vi "Example_OE1022D Control.vi"() -> ()   [LabVIEW 2019]
uses:
  <vilib>/Utility/error.llb/DialogType.ctl
panel:
  in  "Sample count":u32
  out "Zero Data?":bool
  in  "buffer":u8
  out "Queue out":errorcluster caption="error out"
  out "Queue output":refnum<queue>
  in  "Timeout":u32=1000
  out "A_Gain Overlaod":bool
  out "B_Gain Overlaod":bool
  out "B_Input Overlaod":bool
  out "B_PLL Lock":bool
  out "B_Freq":dbl
  out "B_xita":dbl
  out "B_R":dbl
  in  "Remote Mode":u16(ring) items=["USB", "RS232", "GPIB"]
  out "A_Freq":dbl
  out "A_xita":dbl
  out "A_R":dbl
  out "A_Input Overlaod":bool
  out "A_PLL Lock":bool
  out "Error":string
  out "Serial Versions":string
  in  "Table":T1(tab) caption="选项卡控件"
  in  "OE1022D_Configure Input Filter":T2={"Input Source"=0, "Input Shield Grounding "=0, "Input Coupling "=0, "Input Notch Filter "=0, "Channel"=1} {"Channel" items=["A"=1, "B"=2]; "Input Notch Filter" items=["None"=0, "50Hz"=1, "100Hz"=3, "Both"=2]; "Input Coupling" items=["AC", "DC"]; "Input Shield Grounding" items=["Float", "Ground"]; "Input Source" items=["A", "B", "I-1M", "I-100M"]}
  in  "OE1022D_Configure Ref Phase":T3={"Sweep Mode"=0, "Start Frequency"=1000.0, "Stop Frequency"=0.001, "Linear Step Frequency"=1000.0, "Log Step Percent"=10.0, "Step Time(ms)"=1000, "Sweep Run Mode"=0, "Internal Frequency"=1000.0, "Phase  (degree)"=0.0, "External Ref Trigger"=0, "Reference Source"=0, "Channel"=1} {"Channel" items=["A"=1, "B"=2]; "Reference Source" items=["External", "Internal", "Internal Sweep", "Channel-A"]; "External Ref Trigger" items=["TTL Rising Edge", "TTL Falling Edge", "Sine Zero Crossing"]; "Phase  (degree)" min=-180.0 max=180.0 format="%#.2g"; "Internal Frequency" min=0.001 max=102000.0 format="%#.3f"; "Sweep Run Mode" items=["Stop", "Singal", "Loop"]; "Step Time(ms)" min=1 max=100000; "Log Step Percent" min=0.0 max=100.0 format="%#.2g"; "Linear Step Frequency" min=0.001 max=102000.0 format="%#.3f"; "Stop Frequency" min=0.001 max=102000.0 format="%#.3f"; "Start Frequency" min=0.001 max=102000.0 format="%#.3f"; "Sweep Mode" items=["Linear", "Log"]}
  in  "OE1022D_Configure Sens and Filter":T4={"Dynamic Reserve"=1, "Sensitivity "=24, "Time Constant "=9, "Low Pass Filter Slope "=1, "Enable Sync Filter "=0, "Channel"=1} {"Channel" items=["A"=1, "B"=2]; "Enable Sync Filter" items=["OFF", "ON"]; "Low Pass Filter Slope" items=["6 dB/oct", "12 dB/oct", "18 db/oct", "24 dB/oct"]; "Time Constant" items=["10 us", "30 us", "100 us", "300 us", "1 ms", "3 ms", "10 ms", "30 ms", "100 ms", "300 ms", "1 s", "3 s", "10 s", "30 s", "100 s", "300 s", "1 ks", "3 ks"]; "Sensitivity" items=["1 nV/fA", "2 nV/fA", "5 nV/fA", "10 nV/fA", "20 nV/fA", "50 nV/fA", "100 nV/fA", "200 nV/fA", "500 nV/fA", "1 uV/pA", "2 uV/pA", "5 uV/pA", "10 uV/pA", "20 uV/pA", "50 uV/pA", "100 uV/pA", "200 uV/pA", "500 uV/pA", "1 mV/nA", "2 mV/nA", "5 mV/nA", "10 mV/nA", "20 mV/nA", "50 mV/nA", "100 mV/nA", "200 mV/nA", "500 mV/nA", "1 V/uA"]; "Dynamic Reserve" items=["Low Noise", "Normal", "High Reserve"]}
  in  "OE1022D_Configure Channel Out":T5={"CH1 Speed"=0, "CH2 Offset(%)"=0.0, "CH1 Offset(%)"=0.0, "CH2 Expand"=1.0, "CH1 Expand"=1.0, "CH1"=0, "CH2"=0, "AUX OUT1"=1.0, "AUX OUT2"=1.0, "CH2 Speed"=0} {"CH2 Speed" items=["Slow", "Fast"]; "AUX OUT2" min=-10.0 max=10.0 format="%#.3g"; "AUX OUT1" min=-10.0 max=10.0 format="%#.3g"; "CH2" items=["A-R", "A-X", "A-Y", "A-Theta", "A-Rh1", "A-Xh1", "A-Yh1", "A-Theta h1", "A-Rh2", "A-Xh2", "A-Yh2", "A-Theta h2", "A-Noise", "A-E1", "A-E2", "A-E3", "A-E4", "B-R", "B-X", "B-Y", "B-Theta", "B-Rh1", "B-Xh1", "B-Yh1", "B-Theta h1", "B-Rh2", "B-Xh2", "B-Yh2", "B-Theta h2", "B-Noise", "B-E1", "B-E2", "B-E3", "B-E4", "AUX OUT"]; "CH1" items=["A-R", "A-X", "A-Y", "A-Theta", "A-Rh1", "A-Xh1", "A-Yh1", "A-Theta h1", "A-Rh2", "A-Xh2", "A-Yh2", "A-Theta h2", "A-Noise", "A-E1", "A-E2", "A-E3", "A-E4", "B-R", "B-X", "B-Y", "B-Theta", "B-Rh1", "B-Xh1", "B-Yh1", "B-Theta h1", "B-Rh2", "B-Xh2", "B-Yh2", "B-Theta h2", "B-Noise", "B-E1", "B-E2", "B-E3", "B-E4", "AUX OUT"]; "CH1 Expand" min=1.0 max=256.0 format="%#_3g"; "CH2 Expand" min=1.0 max=256.0 format="%#_3g"; "CH1 Offset(%)" min=-100.0 max=100.0 format="%#_5g"; "CH2 Offset(%)" min=-100.0 max=100.0 format="%#_5g"; "CH1 Speed" items=["Slow", "Fast"]}
  in  "OE1022D_Configure Sine Out":T6={"Start Value"=1.0, "Sine Output Amplitude "=1.0, "Stop Valve"=5.0, "Sine Step Valve"=1.0, "Step Time "=1000, "Sine Step Percent"=10.0, "SineOut Mode"=0, "Sine Run Mode"=0, "Channel"=1, "Sine Output DC "=1.0} {"Sine Output DC" min=-10.0 max=10.0 format="%#.3f"; "Channel" items=["A"=1, "B"=2]; "Sine Run Mode" items=["Stop", "Single", "Loop"]; "SineOut Mode" items=["Fixed", "Linear", "Log", "DC"]; "Sine Step Percent" min=0.0 max=100.0 format="%#.3g"; "Step Time" min=1 max=100000; "Sine Step Valve" min=0.001 max=5.0 format="%#.3g"; "Stop Valve" min=0.001 max=5.0 format="%#.3g"; "Sine Output Amplitude" min=0.001 max=5.0 format="%#.3g"; "Start Value" min=0.001 max=5.0 format="%#.3g"}
  in  "OE1022D_Configure Harmonic":T7={"Harmonic 1"=1, "Harmonic 2"=1, "Channel"=1} {"Channel" items=["A"=1, "B"=2]; "Harmonic 2" min=1 max=32767; "Harmonic 1" min=1 max=32767}
  in  "OE1022D_Configure Sample":T8={"Trigger Mode"=0, "Sample Mode"=0, "Buffer 1"=0, "Buffer 2"=1, "Buffer 3"=2, "Sample Time(ms)"=100, "Length"=50, "Buffer 4"=3, "Channel"=1, "Sample State"=0} {"Sample State" items=["Start", "Pause", "Stop and Clear"]; "Channel" items=["A"=1, "B"=2]; "Buffer 4" items=["R", "X", "Y", "Theta", "Rh1", "Xh1", "Yh1", "Theta h1", "Rh2", "Xh2", "Yh2", "Theta h2", "Noise", "A1", "A2", "A3", "A4", "Freq", "C1", "C2"]; "Length" min=1 max=16384; "Sample Time(ms)" min=1 max=100000; "Buffer 3" items=["R", "X", "Y", "Theta", "Rh1", "Xh1", "Yh1", "Theta h1", "Rh2", "Xh2", "Yh2", "Theta h2", "Noise", "A1", "A2", "A3", "A4", "Freq", "C1", "C2"]; "Buffer 2" items=["R", "X", "Y", "Theta", "Rh1", "Xh1", "Yh1", "Theta h1", "Rh2", "Xh2", "Yh2", "Theta h2", "Noise", "A1", "A2", "A3", "A4", "Freq", "C1", "C2"]; "Buffer 1" items=["R", "X", "Y", "Theta", "Rh1", "Xh1", "Yh1", "Theta h1", "Rh2", "Xh2", "Yh2", "Theta h2", "Noise", "A1", "A2", "A3", "A4", "Freq", "C1", "C2"]; "Sample Mode" items=["Single", "Loop"]; "Trigger Mode" items=["Int", "Ext"]}
  in  "OE1022D_Configure Equation":T9={"A"=0, "B"=18, "C"=19, "E"=1, "C1"=0.0, "C2"=0.0, "Channel"=1} {"Channel" items=["A"=1, "B"=2]; "C2" min=-10.0 max=10.0 format="%.3f"; "C1" min=-10.0 max=10.0 format="%.3f"; "E" items=["1"=1, "2"=2, "3"=3, "4"=4]; "C" items=["R", "X", "Y", "Theta", "Rh1", "Xh1", "Yh1", "Theta h1", "Rh2", "Xh2", "Yh2", "Theta h2", "Noise", "A1", "A2", "A3", "A4", "Freq", "C1", "C2"]; "B" items=["R", "X", "Y", "Theta", "Rh1", "Xh1", "Yh1", "Theta h1", "Rh2", "Xh2", "Yh2", "Theta h2", "Noise", "A1", "A2", "A3", "A4", "Freq", "C1", "C2"]; "A" items=["R", "X", "Y", "Theta", "Rh1", "Xh1", "Yh1", "Theta h1", "Rh2", "Xh2", "Yh2", "Theta h2", "Noise", "A1", "A2", "A3", "A4", "Freq", "C1", "C2"]}
  in  "OE1022D_Auto Setting":T10={"Auto Gain"=FALSE, "Auto Reserve"=FALSE, "Auto Phase"=FALSE, "Auto Scale"=FALSE, "Channel"=1} {"Channel" items=["A"=1, "B"=2]}
  in  "Save Button":bool
  in  "file path":path
  in  "Sample Rate":dbl=0.1 min=0.1 max=100.0
  out "Status":string
  in  "Connect":bool
  in  "VISA resource name":refnum<visa-resource-name>
  in  "Baud rate (921600)":u32=921600
  # "Tel          :   +86-020-84133345\nWebsite  :   www.ssi-instrument.com\nE-mail     :   support@si-instrument.com"
  # "X"
  # "="
  # "______________________________________________________"
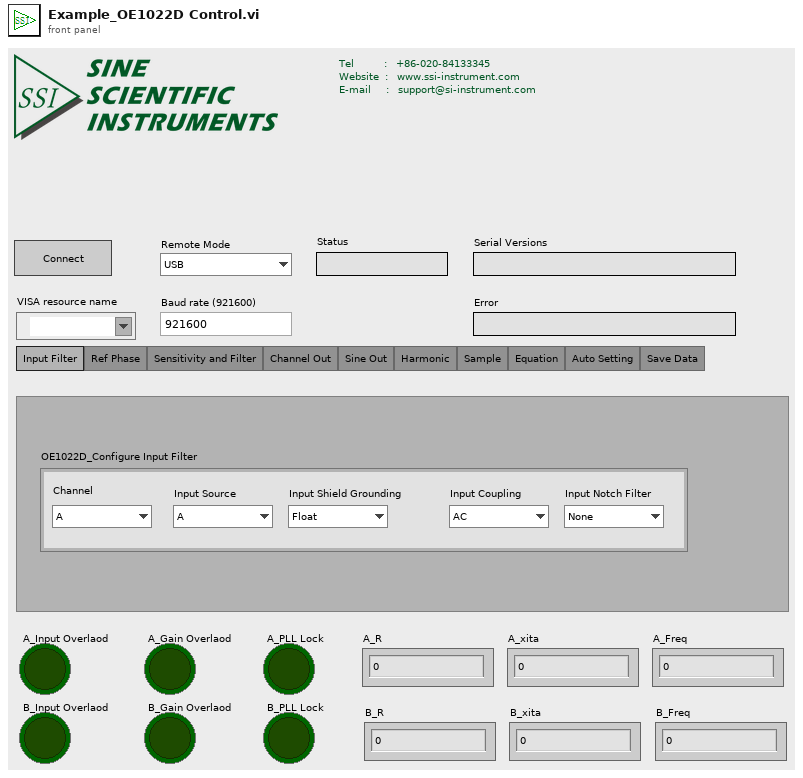
[diagram p1: front panel]
types:
  T1 = enum32{"Input Filter", "Ref Phase", "Sensitivity and Filter", "Channel Out", "Sine Out", "Harmonic", "Sample", "Equation", "Auto Setting", "Save Data"}
  T2 = cluster{"Input Source":u16, "Input Shield Grounding ":u16, "Input Coupling ":u16, "Input Notch Filter ":u16, "Channel":u16}
  T3 = cluster{"Sweep Mode":u16, "Start Frequency":dbl, "Stop Frequency":dbl, "Linear Step Frequency":dbl, "Log Step Percent":dbl, "Step Time(ms)":u32, "Sweep Run Mode":u16, "Internal Frequency":dbl, "Phase  (degree)":dbl, "External Ref Trigger":u16, "Reference Source":u16, "Channel":u16}
  T4 = cluster{"Dynamic Reserve":u16, "Sensitivity ":u16, "Time Constant ":u8, "Low Pass Filter Slope ":u8, "Enable Sync Filter ":u16, "Channel":u16}
  T5 = cluster{"CH1 Speed":u16, "CH2 Offset(%)":dbl, "CH1 Offset(%)":dbl, "CH2 Expand":dbl, "CH1 Expand":dbl, "CH1":u16, "CH2":u16, "AUX OUT1":dbl, "AUX OUT2":dbl, "CH2 Speed":u16}
  T6 = cluster{"Start Value":dbl, "Sine Output Amplitude ":dbl, "Stop Valve":dbl, "Sine Step Valve":dbl, "Step Time ":u32, "Sine Step Percent":dbl, "SineOut Mode":u8, "Sine Run Mode":u8, "Channel":u16, "Sine Output DC ":dbl}
  T7 = cluster{"Harmonic 1":u16, "Harmonic 2":u16, "Channel":u16}
  T8 = cluster{"Trigger Mode":u16, "Sample Mode":u16, "Buffer 1":u16, "Buffer 2":u16, "Buffer 3":u16, "Sample Time(ms)":u32, "Length":u16, "Buffer 4":u16, "Channel":u16, "Sample State":u16}
  T9 = cluster{"A":u16, "B":u16, "C":u16, "E":u16, "C1":dbl, "C2":dbl, "Channel":u16}
  T10 = cluster{"Auto Gain":bool, "Auto Reserve":bool, "Auto Phase":bool, "Auto Scale":bool, "Channel":u16}
  T11 = enum16{"OE1022", "OE1022D", "OE1201", "OE2031&OE2041", "OE1311&OE1351"}
  T12 = cluster{"PLL Lock(1: External Lock)":bool, "Input Overlaod":bool, "Gain Overlaod":bool}
  T13 = cluster{"A_X":dbl, "A_Y":dbl, "A_R":dbl, "A_θ":dbl, "A_Frequency":dbl, "A_Noise":dbl, "A_Xh1":dbl, "A_Yh1":dbl, "A_Rh1":dbl, "A_θh1":dbl, "A_Xh2":dbl, "A_Yh2":dbl, "A_Rh2":dbl, "A_θh2":dbl, "B_X":dbl, "B_Y":dbl, "B_R":dbl, "B_θ":dbl, "B_Frequency":dbl, "B_Noise":dbl, "B_Xh1":dbl, "B_Yh1":dbl, "B_Rh1":dbl, "B_θh1":dbl, "B_Xh2":dbl, "B_Yh2":dbl, "B_Rh2":dbl, "B_θh2":dbl, "A1":dbl, "A2":dbl, "A3":dbl, "A4":dbl}
  T14 = cluster{"A_PLL&Overload":cluster{"PLL Lock(1: External Lock)":bool, "Input Overlaod":bool, "Gain Overlaod":bool}, "B_PLL&Overload":cluster{"PLL Lock(1: External Lock)":bool, "Input Overlaod":bool, "Gain Overlaod":bool}}
  T15 = typedef "DialogType.ctl" = u16
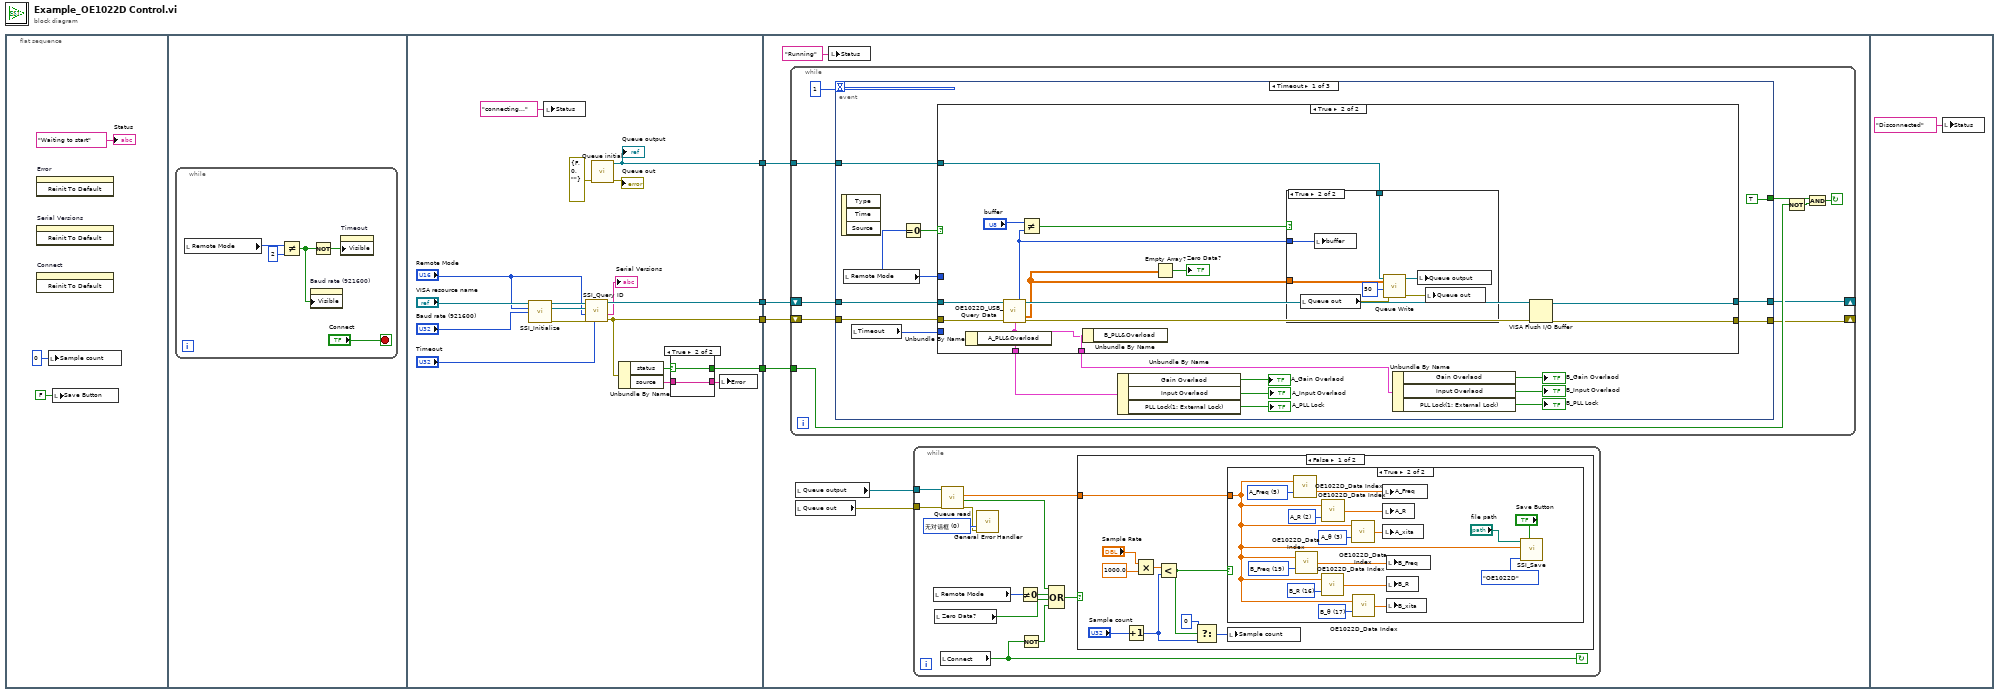
[diagram p0: block diagram]
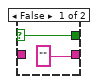
[diagram p2: hidden frame]
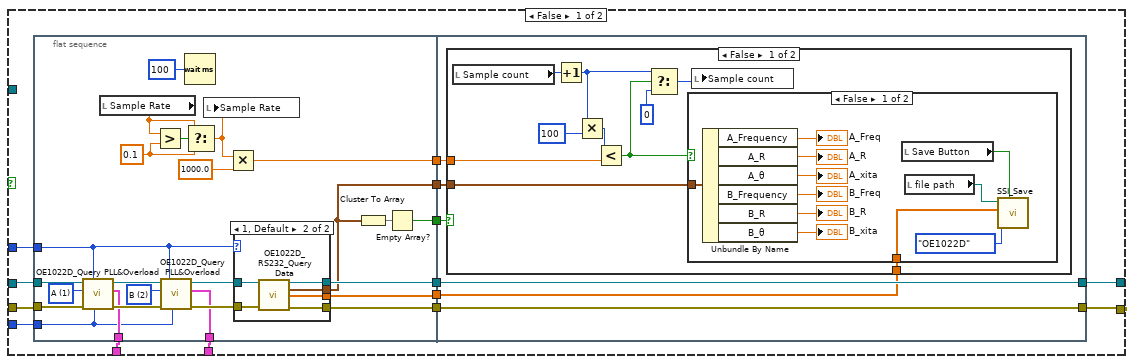
[diagram p5: hidden frame]
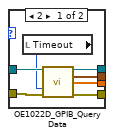
[diagram p6: hidden frame]
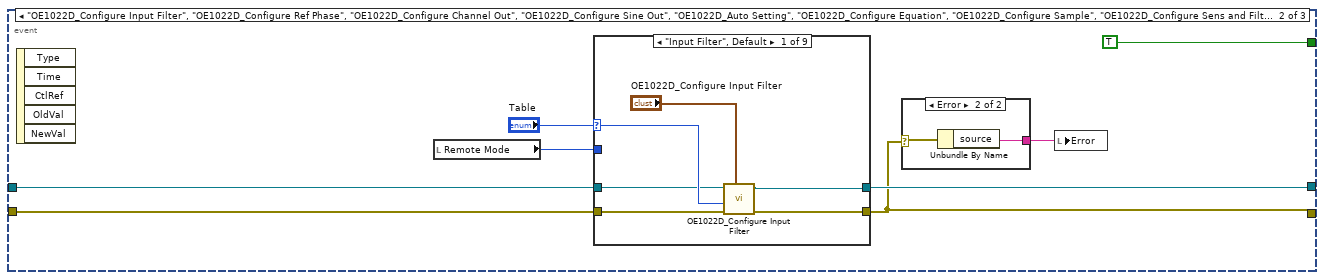
[diagram p10: hidden frame]
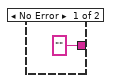
[diagram p11: hidden frame]
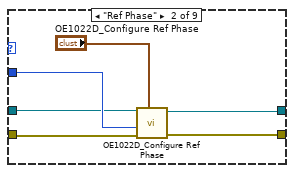
[diagram p12: hidden frame]
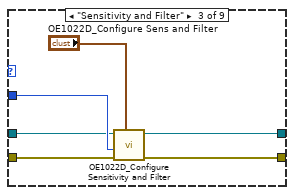
[diagram p13: hidden frame]
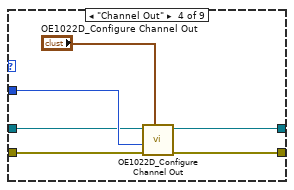
[diagram p14: hidden frame]
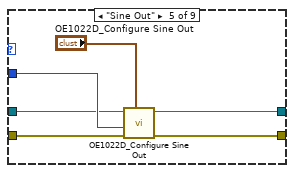
[diagram p15: hidden frame]
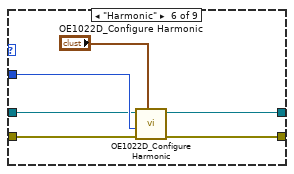
[diagram p16: hidden frame]
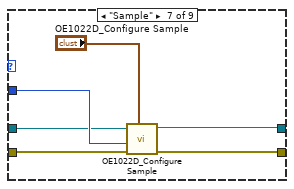
[diagram p17: hidden frame]
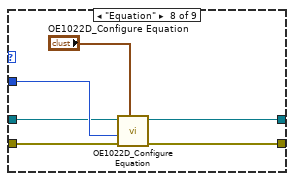
[diagram p18: hidden frame]
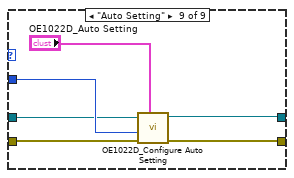
[diagram p19: hidden frame]
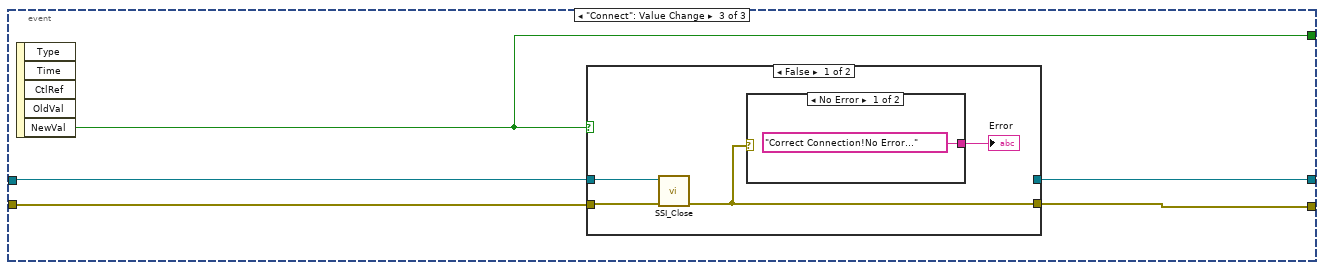
[diagram p20: hidden frame]
diagram:
  n1 = flat-sequence {
    tunnel: [w24] -> w4
    tunnel: [w19] -> w3
    tunnel: [w18] -> w2
    tunnel: [w13] -> w1
    tunnel: w4 -> [w40]
    tunnel: w3 -> [w39]
    tunnel: w2 -> [w38]
    tunnel: w1 -> [w37]
    frame #0 {
      n2 = invoke on="Error" class="Str" method="Reinit To Default"() -> ()  [unwired: 3 in, 3 out]
      n3 = invoke on="Serial Versions" class="Str" method="Reinit To Default"() -> ()  [unwired: 3 in, 3 out]
      n4 = invoke on="Connect" class="Bool (严格)" method="Reinit To Default"() -> ()  [unwired: 3 in, 3 out]
      n5 = local write "Sample count"(u32 0 ("Sample count")) -> ()
      n6 = local write "Save Button"(FALSE ("Save Button")) -> ()
      "Status" <- "Waiting to start" ("status")
    }
    frame #1 {
      n7 = while {
        stop <- "Connect" stop-if-true
        n8 = local read "Remote Mode"() -> (w11:u16)
        n9 = Not Equal?(x=w11, y=u16 2) -> (x != y?=w9:bool)
        n10 = property on="Baud rate (921600)" class="DigNum (strict)"("Visible"=w9) -> ()  [unwired: 2 in, 2 out]
        n11 = Not(x=w9) -> (.not. x?=w8:bool)
        n12 = property on="Timeout" class="DigNum (strict)"("Visible"=w8) -> ()  [unwired: 2 in, 2 out]
      }
    }
    frame #2 {
      n13 = call "SSI_Initialize.vi"("VISA resource name"="VISA resource name", "Remote Mode"="Remote Mode", "baud rate (921600)"="Baud rate (921600)") -> ("VISA resource name out"=w28:refnum<visa-resource-name>, "connection ID(Ethernet)"=w27:refnum<k5>, "error out"=w26:errorcluster)  [unwired: 10 in]
      n14 = local write "Status"("connecting..." ("status")) -> ()
      n15 = call "SSI_Query ID.vi"("Timeout"="Timeout", "Error in (no error)"=w26, "Remote Mode"="Remote Mode", "Connection ID in"=w27, "VISA resource name"=w28) -> ("Error out"=w19:errorcluster, "Read Buffer"=→"Serial Versions":string, "VISA resource  out"=w24:refnum<visa-resource-name>)  [unwired: 3 in, 1 out]
      n16 = call "Queue initial.vi"("Error in (no error)"=errorcluster {"status"=FALSE, "code"=0, "source"=""}) -> ("Error out"=→"Queue out":errorcluster, "Queue output"=w13:refnum<queue>)  [unwired: 9 in]
      "Queue output" <- w13
      n17 = Unbundle By Name(w19) -> ("status"=w21:bool, "source"=w20:string)
      n18 = case shown="True" w21 {
        selector: w21 -> [w32 w34]
        tunnel: [w32 w34] -> w18
        tunnel: ["" w33] -> w17
        tunnel: w20 -> [_ w33]
        frame False {
        }
        frame True {
        }
      }
      n19 = local write "Error"(w17) -> ()
    }
    frame #3 {
      n20 = while {
        tunnel: w38 -> [w82]
        tunnel: w37 -> [w81]
        shift-right: [w79] -> _
        shift-left: w40 -> [w84]
        shift-right: [w80] -> _
        shift-left: w39 -> [w83]
        stop <- w86 continue-if-true
        n21 = event shown="[0] Timeout" {
          selector: _ -> [_ _ _]
          dyn-events: _ -> [_ _ _]
          timeout: 1 -> [_ _ _]
          tunnel: [TRUE ("Stop") TRUE ("Stop") w275] -> w85
          tunnel: [w105 w210 w276] -> w80
          tunnel: [w104 w213 w272] -> w79
          tunnel: w84 -> [w102 w208 w273]
          tunnel: w83 -> [w101 w207 w274]
          tunnel: w81 -> [w90 _ _]
          event Timeout {
            n22 = event-data() -> ()  [unwired: 1 in, 3 out]
            n23 = local read "Remote Mode"() -> (w92:u16)
            n24 = local read "Timeout"() -> (w89:u32)
            n25 = Equal To 0?(x=w92) -> (x = 0?=w91:bool)
            n26 = case shown="True" w91 {
              tunnel: [w119 w186] -> w105
              tunnel: [w118 w187] -> w104
              tunnel: w102 -> [w117 w192]
              tunnel: w101 -> [w116 w191]
              tunnel: [w115 w190] -> w100
              tunnel: [w114 w189] -> w99
              tunnel: w92 -> [w113 _]
              tunnel: w90 -> [_ w185]
              tunnel: w89 -> [w106 _]
              frame False {
                n27 = flat-sequence {
                  tunnel: [w131] -> w112
                  tunnel: [w132] -> w111
                  tunnel: [w140] -> w109
                  tunnel: [w122] -> w108
                  tunnel: [w130] -> w107
                  tunnel: [w127] -> w115
                  tunnel: [w126] -> w114
                  tunnel: w117 -> [w129]
                  tunnel: w116 -> [w128]
                  tunnel: w113 -> [w125]
                  tunnel: [w123] -> w110
                  tunnel: w106 -> [w120]
                  tunnel: w112 -> [w162]
                  tunnel: w111 -> [w163]
                  tunnel: [w163] -> w118
                  tunnel: [w162] -> w119
                  tunnel: w110 -> [w159]
                  tunnel: w109 -> [w158]
                  tunnel: w108 -> [w160]
                  tunnel: w107 -> [w161]
                  frame #0 {
                    w136 = u16 2 items=["A"=1, "B"=2] ("Channel")
                    w137 = u16 1 items=["A"=1, "B"=2] ("Channel")
                    w143 = 0.1 ("y")
                    n28 = call "OE1022D_Query PLL&Overload.vi"("Timeout"=w120, "Error in (no error)"=w128, "Remote Mode"=w125, "Channel"=w137, "VISA resource name"=w129) -> ("Error out"=w138:errorcluster, "OE1022D_Query PLL&Overload"=w127:T12, "VISA resource  out"=w135:refnum<visa-resource-name>)  [unwired: 3 in, 1 out]
                    n29 = local read "Sample Rate"() -> (w139:dbl)
                    n30 = Greater?(x=w139, y=w143) -> (0:w142:bool)
                    n31 = call "OE1022D_Query PLL&Overload.vi"("Timeout"=w120, "Error in (no error)"=w138, "Remote Mode"=w125, "Channel"=w136, "VISA resource name"=w135) -> ("Error out"=w134:errorcluster, "OE1022D_Query PLL&Overload"=w126:T12, "VISA resource  out"=w133:refnum<visa-resource-name>)  [unwired: 3 in, 1 out]
                    n32 = Wait (ms)(milliseconds to wait=u32 100 ("等待时间（毫秒）")) -> ()  [unwired: 1 out]
                    n33 = Select(t=w139, s=w142, f=w143) -> (s? t:f=w141:dbl)
                    n34 = local write "Sample Rate"(w141) -> ()
                    n35 = Multiply(x=w141, y=1000.0) -> (x*y=w140:dbl)
                    n36 = case shown="1, Default" w125 {
                      tunnel: w134 -> [w150 w157]
                      tunnel: w133 -> [w151 w156]
                      tunnel: [w149 w155] -> w132
                      tunnel: [w148 w154] -> w131
                      tunnel: [w147 w153] -> w130
                      tunnel: [w146 w152] -> w122
                      frame 2 {
                        n37 = local read "Timeout"() -> (w145:u32)
                        n38 = call "OE1022D_GPIB_Query Data.vi"("VISA resource name"=w151, "Timeout"=w145, "Error in (no error)"=w150) -> ("VISA resource  out"=w149:refnum<visa-resource-name>, "Parameter Values"=w146:T13, "Data Array"=w147:dbl[], "Error out"=w148:errorcluster)  [unwired: 8 in, 1 out]
                      }
                      frame 1, Default {
                        n39 = call "OE1022D_RS232_Query Data.vi"("VISA resource name"=w156, "Error in (no error)"=w157) -> ("VISA resource  out"=w155:refnum<visa-resource-name>, "Parameter Values"=w152:T13, "Data Array"=w153:dbl[], "Error out"=w154:errorcluster)  [unwired: 9 in, 1 out]
                      }
                    }
                    n40 = Cluster To Array(cluster=w122) -> (array=w124:dbl[])
                    n41 = Empty Array?(array=w124) -> (empty?=w123:bool)
                  }
                  frame #1 {
                    n42 = case shown="False" w159 {
                      tunnel: w161 -> [w173 _]
                      tunnel: w160 -> [w172 _]
                      tunnel: w158 -> [w168 _]
                      frame False {
                        n43 = local read "Sample count"() -> (w171:u32)
                        n44 = Increment(x=w171) -> (x+1=w167:u32)
                        n45 = Multiply(x=w167, y=u32 100) -> (x*y=w169:u32)
                        n46 = Less?(x=w169, y=w168) -> (x < y?=w165:bool)
                        n47 = Select(t=w167, s=w165, f=0) -> (s? t:f=w166:u32)
                        n48 = case shown="False" w165 {
                          tunnel: w172 -> [w175 _]
                          tunnel: w173 -> [w184 _]
                          frame False {
                            n49 = Unbundle By Name(w175) -> ("A_Frequency"=→"A_Freq":dbl, "A_R"=→"A_R":dbl, "A_θ"=→"A_xita":dbl, "B_Frequency"=→"B_Freq":dbl, "B_R"=→"B_R":dbl, "B_θ"=→"B_xita":dbl)
                            n50 = local read "Save Button"() -> (w182:bool)
                            n51 = local read "file path"() -> (w174:path)
                            n52 = call "SSI_Save.vi"("file path (dialog if empty)"=w174, "1D data"=w184, "Instrument Mode"=T11."OE1022D", "Save Button"=w182) -> ()  [unwired: 7 in]
                          }
                          frame True {
                          }
                        }
                        n53 = local write "Sample count"(w166) -> ()
                      }
                      frame True {
                      }
                    }
                  }
                }
              }
              frame True {
                n54 = call "OE1022D_USB_Query Data.vi"("VISA resource name"=w192, "Error in (no error)"=w191) -> ("Buffer Count"=w193:u8, "VISA resource  out"=w199:refnum<visa-resource-name>, "Total Date Array"=w194:dbl[][], "PLL&Overload"=w188:T14, "Error out"=w198:errorcluster)  [unwired: 6 in, 3 out]
                n55 = Unbundle By Name(w188) -> ("A_PLL&Overload"=w190:T12)
                n56 = Not Equal?(x="buffer", y=w193) -> (x != y?=w196:bool)
                n57 = Unbundle By Name(w188) -> ("B_PLL&Overload"=w189:T12)
                n58 = Empty Array?(array=w194) -> (empty?=→"Zero Data?":bool)
                n59 = case shown="True" w196 {
                  tunnel: w194 -> [_ w202]
                  tunnel: w193 -> [_ w201]
                  tunnel: w185 -> [_ w200]
                  frame False {
                  }
                  frame True {
                    n60 = local read "Queue out"() -> (w203:errorcluster)
                    n61 = local write "buffer"(w201) -> ()
                    n62 = call "Queue Write.vi"("Error in (no error)"=w203, "Group Count"=50, "Input Array"=w202, "Queue Input"=w200) -> ("Error out"=w204:errorcluster, "Queue output"=w205:refnum<queue>)  [unwired: 6 in]
                    n63 = local write "Queue output"(w205) -> ()
                    n64 = local write "Queue out"(w204) -> ()
                  }
                }
                n65 = VISA Flush I/O Buffer(VISA resource name=w199, error in (no error)=w198) -> (VISA resource name out=w187:refnum<visa-resource-name>, error out=w186:errorcluster)  [unwired: 1 in]
              }
            }
            n66 = Unbundle By Name(w100) -> ("Gain Overlaod"=→"A_Gain Overlaod":bool, "Input Overlaod"=→"A_Input Overlaod":bool, "PLL Lock(1: External Lock)"=→"A_PLL Lock":bool)
            n67 = Unbundle By Name(w99) -> ("Gain Overlaod"=→"B_Gain Overlaod":bool, "Input Overlaod"=→"B_Input Overlaod":bool, "PLL Lock(1: External Lock)"=→"B_PLL Lock":bool)
          }
          event "OE1022D_Configure Input Filter", "OE1022D_Configure Ref Phase", "OE1022D_Configure Channel Out", "OE1022D_Configure Sine Out", "OE1022D_Auto Setting", "OE1022D_Configure Equation", "OE1022D_Configure Sample", "OE1022D_Configure Sens and Filter", "OE1022D_Configure Harmonic": Value Change {
            n68 = event-data() -> ()  [unwired: 1 in, 5 out]
            n69 = local read "Remote Mode"() -> (w211:u16)
            n70 = case shown="\"Input Filter\", Default" "Table" {
              selector: "Table" -> [w223 _ _ _ _ _ _ _ _]
              tunnel: [w221 w228 w234 w240 w246 w251 w259 w262 w269] -> w213
              tunnel: [w220 w227 w235 w239 w247 w252 w258 w265 w268] -> w210
              tunnel: w211 -> [_ w226 w232 w238 w244 w250 w257 w264 w270]
              tunnel: w208 -> [w219 w225 w231 w237 w243 w249 w255 w261 w267]
              tunnel: w207 -> [w218 w224 w230 w236 w242 w248 w254 w260 w266]
              frame "Input Filter", Default {
                n71 = call "OE1022D_Configure Input Filter.vi"("OE1022D_Configure Input Filter"="OE1022D_Configure Input Filter", "Error in (no error)"=w218, "Remote Mode"=w223, "VISA resource name"=w219) -> ("Error out"=w220:errorcluster, "VISA resource  out"=w221:refnum<visa-resource-name>)  [unwired: 5 in, 1 out]
              }
              frame "Ref Phase" {
                n72 = call "OE1022D_Configure Ref Phase.vi"("OE1022D_Configure Ref Phase"="OE1022D_Configure Ref Phase", "Error in (no error)"=w224, "Remote Mode"=w226, "VISA resource name"=w225) -> ("Error out"=w227:errorcluster, "VISA resource  out"=w228:refnum<visa-resource-name>)  [unwired: 5 in, 1 out]
              }
              frame "Sensitivity and Filter" {
                n73 = call "OE1022D_Configure Sensitivity and Filter.vi"("OE1022D_Configure Sens and Filter"="OE1022D_Configure Sens and Filter", "Error in (no error)"=w230, "Remote Mode"=w232, "VISA resource name"=w231) -> ("Error out"=w235:errorcluster, "VISA resource  out"=w234:refnum<visa-resource-name>)  [unwired: 5 in, 1 out]
              }
              frame "Channel Out" {
                n74 = call "OE1022D_Configure Channel Out.vi"("OE1022D_Configure Channel Out"="OE1022D_Configure Channel Out", "Error in (no error)"=w236, "Remote Mode"=w238, "VISA resource name"=w237) -> ("Error out"=w239:errorcluster, "VISA resource  out"=w240:refnum<visa-resource-name>)  [unwired: 5 in, 1 out]
              }
              frame "Sine Out" {
                n75 = call "OE1022D_Configure Sine Out.vi"("OE1022D_Configure Sine Out"="OE1022D_Configure Sine Out", "Error in (no error)"=w242, "Remote Mode"=w244, "VISA resource name"=w243) -> ("Error out"=w247:errorcluster, "VISA resource  out"=w246:refnum<visa-resource-name>)  [unwired: 5 in, 1 out]
              }
              frame "Harmonic" {
                n76 = call "OE1022D_Configure Harmonic.vi"("OE1022D_Configure Harmonic"="OE1022D_Configure Harmonic", "Error in (no error)"=w248, "Remote Mode"=w250, "VISA resource name"=w249) -> ("Error out"=w252:errorcluster, "VISA resource  out"=w251:refnum<visa-resource-name>)  [unwired: 5 in, 1 out]
              }
              frame "Sample" {
                n77 = call "OE1022D_Configure Sample.vi"("OE1022D_Configure Sample"="OE1022D_Configure Sample", "Error in (no error)"=w254, "Remote Mode"=w257, "VISA resource name"=w255) -> ("Error out"=w258:errorcluster, "VISA resource  out"=w259:refnum<visa-resource-name>)  [unwired: 5 in, 1 out]
              }
              frame "Equation" {
                n78 = call "OE1022D_Configure Equation.vi"("OE1022D_Configure Equation"="OE1022D_Configure Equation", "Error in (no error)"=w260, "Remote Mode"=w264, "VISA resource name"=w261) -> ("Error out"=w265:errorcluster, "VISA resource  out"=w262:refnum<visa-resource-name>)  [unwired: 5 in, 1 out]
              }
              frame "Auto Setting" {
                n79 = call "OE1022D_Configure Auto Setting.vi"("OE1022D_Auto Setting"="OE1022D_Auto Setting", "Error in (no error)"=w266, "Remote Mode"=w270, "VISA resource name"=w267) -> ("Error out"=w268:errorcluster, "VISA resource  out"=w269:refnum<visa-resource-name>)  [unwired: 5 in, 1 out]
              }
            }
            n80 = case shown="Error" w210 {
              selector: w210 -> [_ w217]
              tunnel: ["" ("source") w216] -> w209
              frame No Error {
              }
              frame Error {
                n81 = Unbundle By Name(w217) -> ("source"=w216:string)
              }
            }
            n82 = local write "Error"(w209) -> ()
          }
          event "Connect": Value Change {
            n83 = event-data() -> ("NewVal"=w275:bool)  [unwired: 1 in, 4 out]
            n84 = case shown="False" w275 {
              tunnel: [w280 w285] -> w276
              tunnel: w274 -> [w278 w285]
              tunnel: w273 -> [w277 w284]
              tunnel: [_ w284] -> w272
              frame False {
                n85 = call "SSI_Close.vi"("Error in (no error)"=w278, "VISA resource name"=w277) -> ("Error out"=w280:errorcluster)  [unwired: 5 in]
                n86 = case shown="No Error" w280 {
                  selector: w280 -> [_ w283]
                  tunnel: ["Correct Connection!No Error..." ("source") w282] -> w279
                  frame No Error {
                  }
                  frame Error {
                    n87 = Unbundle By Name(w283) -> ("source"=w282:string)
                  }
                }
                "Error" <- w279
              }
              frame True {
              }
            }
          }
        }
        n88 = Not(x=w82) -> (.not. x?=w87:bool)
        n89 = And(x=w85, y=w87) -> (x .and. y?=w86:bool)
      }
      n90 = local read "Queue output"() -> (w36:refnum<queue>)
      n91 = local read "Queue out"() -> (w35:errorcluster)
      n92 = local write "Status"("Running" ("status")) -> ()
      n93 = while {
        tunnel: w36 -> [w44]
        tunnel: w35 -> [w43]
        stop <- w48 continue-if-true
        w47 = T15 0 items=["无对话框", "确定信息", "继续或停止信息", "确定信息＋警告", "继续/停止+警告"] ("type of dialog (OK msg:1)")
        n94 = local read "Remote Mode"() -> (w50:u16)
        n95 = local read "Zero Data?"() -> (w51:bool)
        n96 = local read "Connect"() -> (w48:bool)
        n97 = call "Queue read.vi"("Error in (no error)"=w43, "Queue Input"=w44) -> ("Error out"=w46:errorcluster, "Timeout？"=w42:bool, "Output Array"=w45:sgl[])  [unwired: 7 in]
        n98 = call <vilib>:"General Error Handler.vi"("type of dialog (OK msg:1)"=w47, "error in (no error)"=w46) -> ()  [unwired: 9 in, 5 out]
        n99 = Not Equal To 0?(x=w50) -> (x != 0?=w52:bool)
        n100 = Not(x=w48) -> (.not. x?=w49:bool)
        n101 = Compound Arithmetic op=OR(w42, w52, w51, w49) -> (w53:bool)
        n102 = case shown="False" w53 {
          tunnel: w45 -> [w62 _]
          frame False {
            n103 = Increment(x="Sample count") -> (x+1=w55:u32)
            n104 = Multiply(x="Sample Rate", y=1000.0) -> (x*y=w60:dbl)
            n105 = Less?(x=w60, y=w55) -> (x < y?=w57:bool)
            n106 = Select(t=u32 0 ("Sample count"), s=w57, f=w55) -> (s? t:f=w54:u32)
            n107 = case shown="True" w57 {
              tunnel: w62 -> [_ w65]
              frame False {
              }
              frame True {
                w78 = u16 17 items=["A_X", "A_Y", "A_R", "A_θ", "A_Noise", "A_Freq", "A_XD1", "A_YD1", "A_RD1", "A_θD1", "A_XD2", "A_YD2", "A_RD2", "A_θD2", "B_X", "B_Y", "B_R", "B_θ", "B_Noise", "B_Freq", "B_XD1", "B_YD1", "B_RD1", "B_θD1", "B_XD2", "B_YD2", "B_RD2", "B_θD3", "ADC1", "ADC2", "ADC3", "ADC4"] ("Parameter Type")
                w67 = u16 16 items=["A_X", "A_Y", "A_R", "A_θ", "A_Noise", "A_Freq", "A_XD1", "A_YD1", "A_RD1", "A_θD1", "A_XD2", "A_YD2", "A_RD2", "A_θD2", "B_X", "B_Y", "B_R", "B_θ", "B_Noise", "B_Freq", "B_XD1", "B_YD1", "B_RD1", "B_θD1", "B_XD2", "B_YD2", "B_RD2", "B_θD3", "ADC1", "ADC2", "ADC3", "ADC4"] ("Parameter Type")
                w68 = u16 19 items=["A_X", "A_Y", "A_R", "A_θ", "A_Noise", "A_Freq", "A_XD1", "A_YD1", "A_RD1", "A_θD1", "A_XD2", "A_YD2", "A_RD2", "A_θD2", "B_X", "B_Y", "B_R", "B_θ", "B_Noise", "B_Freq", "B_XD1", "B_YD1", "B_RD1", "B_θD1", "B_XD2", "B_YD2", "B_RD2", "B_θD3", "ADC1", "ADC2", "ADC3", "ADC4"] ("Parameter Type")
                w69 = u16 3 items=["A_X", "A_Y", "A_R", "A_θ", "A_Noise", "A_Freq", "A_XD1", "A_YD1", "A_RD1", "A_θD1", "A_XD2", "A_YD2", "A_RD2", "A_θD2", "B_X", "B_Y", "B_R", "B_θ", "B_Noise", "B_Freq", "B_XD1", "B_YD1", "B_RD1", "B_θD1", "B_XD2", "B_YD2", "B_RD2", "B_θD3", "ADC1", "ADC2", "ADC3", "ADC4"] ("Parameter Type")
                w70 = u16 2 items=["A_X", "A_Y", "A_R", "A_θ", "A_Noise", "A_Freq", "A_XD1", "A_YD1", "A_RD1", "A_θD1", "A_XD2", "A_YD2", "A_RD2", "A_θD2", "B_X", "B_Y", "B_R", "B_θ", "B_Noise", "B_Freq", "B_XD1", "B_YD1", "B_RD1", "B_θD1", "B_XD2", "B_YD2", "B_RD2", "B_θD3", "ADC1", "ADC2", "ADC3", "ADC4"] ("Parameter Type")
                w71 = u16 5 items=["A_X", "A_Y", "A_R", "A_θ", "A_Noise", "A_Freq", "A_XD1", "A_YD1", "A_RD1", "A_θD1", "A_XD2", "A_YD2", "A_RD2", "A_θD2", "B_X", "B_Y", "B_R", "B_θ", "B_Noise", "B_Freq", "B_XD1", "B_YD1", "B_RD1", "B_θD1", "B_XD2", "B_YD2", "B_RD2", "B_θD3", "ADC1", "ADC2", "ADC3", "ADC4"] ("Parameter Type")
                n108 = call "OE1022D_Data Index.vi"("Parameter Type"=w71, "Input Date Array"=w65) -> ("Parameter"=w77:dbl)
                n109 = call "OE1022D_Data Index.vi"("Parameter Type"=w68, "Input Date Array"=w65) -> ("Parameter"=w72:dbl)
                n110 = call "OE1022D_Data Index.vi"("Parameter Type"=w67, "Input Date Array"=w65) -> ("Parameter"=w73:dbl)
                n111 = call "OE1022D_Data Index.vi"("Parameter Type"=w70, "Input Date Array"=w65) -> ("Parameter"=w76:dbl)
                n112 = call "OE1022D_Data Index.vi"("Parameter Type"=w69, "Input Date Array"=w65) -> ("Parameter"=w75:dbl)
                n113 = call "OE1022D_Data Index.vi"("Parameter Type"=w78, "Input Date Array"=w65) -> ("Parameter"=w74:dbl)
                n114 = local write "A_Freq"(w77) -> ()
                n115 = local write "A_R"(w76) -> ()
                n116 = local write "A_xita"(w75) -> ()
                n117 = local write "B_Freq"(w72) -> ()
                n118 = local write "B_R"(w73) -> ()
                n119 = local write "B_xita"(w74) -> ()
                n120 = call "SSI_Save.vi"("file path (dialog if empty)"="file path", "1D data"=w65, "Instrument Mode"=T11."OE1022D", "Save Button"="Save Button") -> ()  [unwired: 7 in]
              }
            }
            n121 = local write "Sample count"(w54) -> ()
          }
          frame True {
          }
        }
      }
    }
    frame #4 {
      n122 = local write "Status"("Disconnected" ("status")) -> ()
    }
  }
